vi "XLP80_Action_BuildMessages.vi"(6 "Init":bool, 8 "err in":errorcluster caption="error", 9 "TimeStamp":dbl format="%.2f") -> (0 "err out":errorcluster caption="error", 2 "Messages":string)   [LabVIEW 2021]
uses:
  XLP80_FGlob/1886_FGlob_TDefs_Enum_FGlobItems.ctl
  XLP80_FGlob/1886_FGlob_TDefEnumCANReadItems.ctl
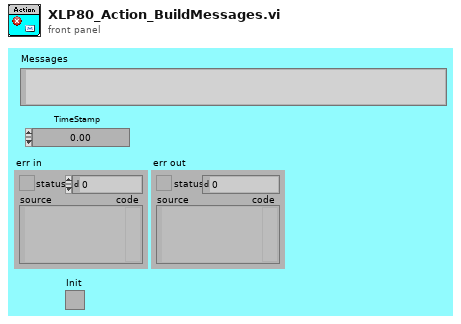
[diagram p1: front panel]
types:
  T1 = typedef "1886_FGlob_TDefEnumCANReadItems.ctl" = enum16{"A03_ETC_a_opCmd1_Start_Stop", "A03_ETC_s_Speed_Actual", "A11_HBV_s_Valve_Act", "A12_SIV_s_Valve_Act", "A13_SOV_s_Valve_Act", "A14_HFM_s_AirMassFlow", "A14_HFM_s_Humidity", "A14_HFM_s_Pressure", "A14_HFM_s_Temperature", "A15_SI_s_Inlet_Pressure", "A15_SI_s_Inlet_Pressure_FM12", "A15_SI_s_Inlet_Temperature", "A16_SI_s_Inlet_Temperature", "A17_SO_s_Outlet_Pressure", "A17_SO_s_Outlet_Pressure_FM12", "A17_SO_s_Outlet_Temperature", "A22_HSI_s_Humidity", "A22_HSI_s_Humidity_FM12", "A23_HSO_s_Humidity", "A56_SO_s_Temperature", "C01_RF_a_FanSpeed", "C02_CP_s_ACTUAL_SPEED_FM2", "C02_CP_a_ENABLE_FM2", "C02_CP_a_RPM", "C04_DI_s_Temperature", "C06_ET_s_CoolLevelStatus", "C07_BAT_s_Board_Temperature", "C07_BAT_s_External_Load_Voltage", "C_07_BAT_s_SoC", "C07_BAT_s_System_Current", "C08_AMB_s_Humidity_Rel", "C08_AMB_s_Pressure", "C08_AMB_s_Temperature", "C24_TRO_s_Temperature_FM23", "C27_RIV_a_Valve_Set_FM2", "C28_RBV_a_Valve_Set_FM2", "C29_TSO_s_Temperature_FM3", "C54_SI_s_Temperature", "C61_SV_a_FanEnable_FM2", "E71_DC4880_s_Current_In_Actual", "E71_DC4880_s_Current_Out_Actual", "E71_DC4880_s_Temperature_1_Act", "E71_DC4880_s_Voltage_Out_Actual", "E71_DC4880_s_Voltage_In_Actual", "E76_HVM_a_Relais_Set", "E75_HVP_a_Relais_Set", "H31_OTV_a_Valve_Set", "H_31_OTV_s_Pressure", "H31_OTV_s_Pressure_FM12", "H_31_OTV_s_Temperature", "H36_GHU_s_Pressure_1", "H36_GHU_s_Pressure_1_FM12", "H37_GHU_s_Temperature_1", "H36_GHU_s_Temperature_FM2", "H38_HSV_a_Valve_Set", "H40_GHU_s_Pressure_2", "H40_GHU_s_Pressure_2_FM12", "H41_GHU_s_Temperature_2", "H42_HRB_s_ARB_Spd", "H43_HDV_a_Dosing_Valve_Set", "H45_WT_s_WaterLevelStatus", "H51_STK_s_CellVolt_highest_2003", "H51_STK_s_CellVolt_lowest_2003", "H51_STK_s_TotalVoltage_2003", "H52_DV_a_Drain_Valve_Stack_Set", "H53_PV_a_Purge_Valve_Stack_Set", "H55_SI_s_Stack_Inlet_Pressure", "H62_HLD_s_H2_Concentration", "H63_HLD_s_H2_Concentration", "H63_HLD_s_concH2_FM2", "S91_SYS_MasterCtrl_State", "S91_SYS_PowerCtrl_State", "S91_SYS_Error_Code", "S91_SYS_Error_Level"}
  T2 = typedef "1886_FGlob_TDefs_Enum_FGlobItems.ctl" = enum16{"Put one", "Put all", "Recall one", "Recall all"}
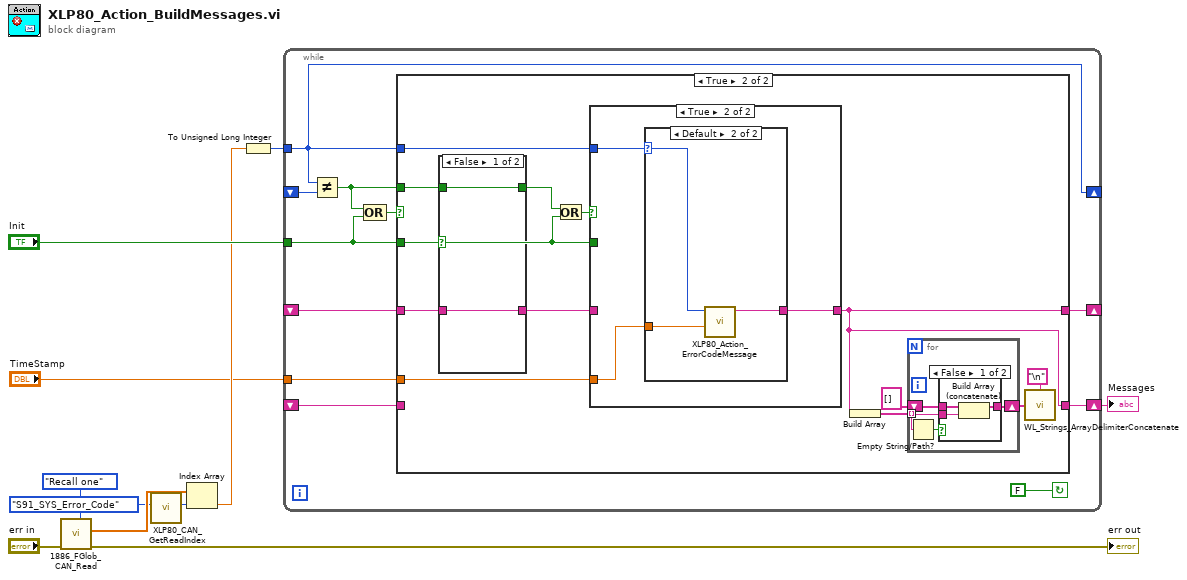
[diagram p0: block diagram]
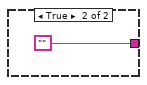
[diagram p4: hidden frame]
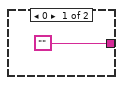
[diagram p5: hidden frame]
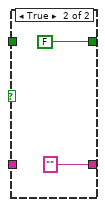
[diagram p6: hidden frame]
diagram:
  n1 = call "1886_FGlob_CAN_Read.vi"("Function (Recall One)"=1886_FGlob_TDefs_Enum_FGlobItems."Recall one", "err in"="err in") -> ("err out"=→"err out":errorcluster, "AI Values OUT"=w8:dbl[])  [unwired: 7 in, 1 out]
  n2 = call "XLP80_CAN_GetReadIndex.vi"("CAN Read Items"=1886_FGlob_TDefEnumCANReadItems."S91_SYS_Error_Code") -> ("Index"=w7:i32)  [unwired: 10 in]
  n3 = Index Array(array=w8, index=w7) -> (element=w3:dbl)
  n4 = To Unsigned Long Integer(number=w3) -> (unsigned 32bit integer=w2:u32)
  n5 = while {
    shift-right: [w16] -> _
    shift-left: _ -> [w14]
    shift-right: [w22] -> _
    shift-left: _ -> [w21]
    shift-right: [w20] -> w11
    shift-left: _ -> [w19]
    tunnel: w2 -> [w16]
    tunnel: "Init" -> [w15]
    tunnel: "TimeStamp" -> [w12]
    stop <- FALSE continue-if-true
    n6 = Not Equal?(x=w16, y=w14) -> (x != y?=w13:bool)
    n7 = Compound Arithmetic op=OR(w13, w15) -> (w17:bool)
    n8 = case shown="True" w17 {
      tunnel: [w23 w26] -> w22
      tunnel: w13 -> [_ w33]
      tunnel: w21 -> [w23 w30]
      tunnel: w16 -> [_ w37]
      tunnel: [w24 w26] -> w20
      tunnel: w15 -> [_ w29]
      tunnel: w19 -> [w24 _]
      tunnel: w12 -> [_ w25]
      frame False {
      }
      frame True {
        n9 = case shown="False" w29 {
          tunnel: w33 -> [w51 _]
          tunnel: [w51 FALSE] -> w32
          tunnel: [w50 ""] -> w31
          tunnel: w30 -> [w50 _]
          frame False {
          }
          frame True {
          }
        }
        n10 = Or(x=w32, y=w29) -> (x .or. y?=w28:bool)
        n11 = case shown="True" w28 {
          tunnel: [w39 w45] -> w26
          tunnel: w37 -> [_ w44]
          tunnel: w31 -> [w40 _]
          tunnel: w29 -> [w38 _]
          tunnel: w25 -> [_ w43]
          frame False {
            n12 = case shown="False" w38 {
              tunnel: w40 -> [w41 _]
              tunnel: [w41 ""] -> w39
              frame False {
              }
              frame True {
              }
            }
          }
          frame True {
            n13 = case shown="Default" w44 {
              selector: w44 -> [_ w48]
              tunnel: ["" w49] -> w45
              tunnel: w43 -> [_ w47]
              frame 0 {
              }
              frame Default {
                n14 = call "XLP80_Action_ErrorCodeMessage.vi"("TimeStamp"=w47, "SYS_Error_Code"=w48) -> ("message string"=w49:string)  [unwired: 9 in]
              }
            }
          }
        }
        n15 = Build Array(w26) -> (w27:string[])
        n16 = for {
          shift-right: [w55] -> w34
          shift-left: string[] [] -> [w56]
          tunnel: w27 -> [w54] mode=indexing
          n17 = Empty String/Path?(string/path=w54) -> (empty?=w57:bool)
          n18 = case shown="False" w57 {
            tunnel: w56 -> [w60 w61]
            tunnel: [w59 w61] -> w55
            tunnel: w54 -> [w58 _]
            frame False {
              n19 = Build Array (concatenate)(w60, w58) -> (w59:string[])
            }
            frame True {
            }
          }
        }
        n20 = call "WL_Strings_ArrayDelimiterConcatenate.vi"("String Array"=w34, "Delimiter (Tab)"="\n") -> ()  [unwired: 1 out]
      }
    }
  }
  "Messages" <- w11
